vi "Przelicz ROS-a.vi"(7 "Vlin multiply":dbl, 8 "angular":dbl format="%#_13g", 9 "linear":dbl format="%#_13g", 10 "Enum":enum16{"LABVIEW", "ROS"}(ring), 11 "szablon CMD_VEL":T1) -> (3 "ROS data converted":cluster{dbl, dbl})   [LabVIEW 2015]
panel:
  in  "ROS data":T2
  out "axes":sgl[](array[numeric])
  out "buttons":i32[](array[numeric])
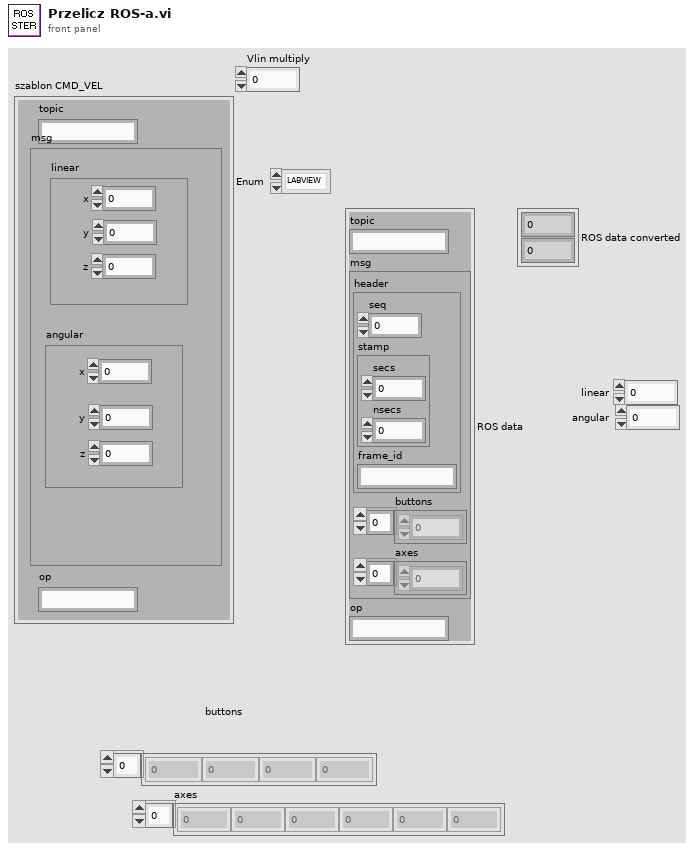
[diagram p1: front panel]
types:
  T1 = cluster{"topic":string, "msg":cluster{"linear":cluster{"x":dbl, "y":dbl, "z":dbl}, "angular":cluster{"x":dbl, "y":dbl, "z":dbl}}, "op":string}
  T2 = cluster{"topic":string, "msg":cluster{"header":cluster{"seq":u32, "stamp":cluster{"secs":u32, "nsecs":i32}, "frame_id":string}, "buttons":i32[], "axes":sgl[]}, "op":string}
  T3 = cluster{"linear":cluster{"x":dbl, "y":dbl, "z":dbl}, "angular":cluster{"x":dbl, "y":dbl, "z":dbl}}
  T4 = cluster{"header":cluster{"seq":u32, "stamp":cluster{"secs":u32, "nsecs":i32}, "frame_id":string}, "buttons":i32[], "axes":sgl[]}
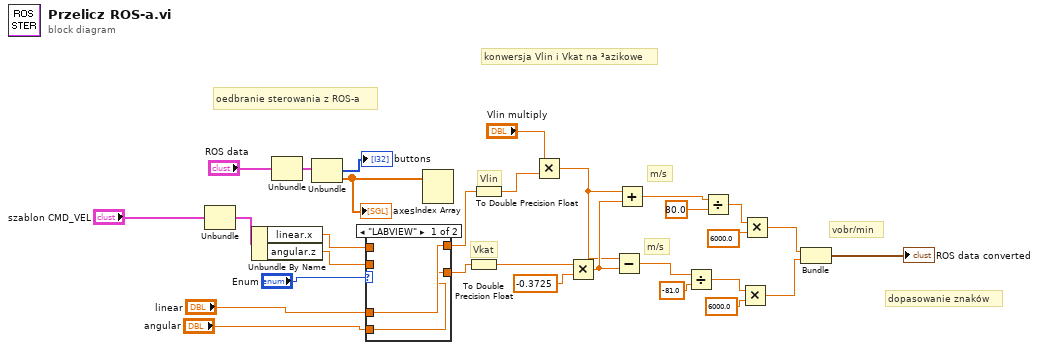
[diagram p0: block diagram]
diagram:
  # "konwersja Vlin i Vkat na ³azikowe"
  # "oedbranie sterowania z ROS-a"
  # "dopasowanie znaków"
  # "vobr/min"
  # "m/s"
  # "m/s"
  # "Vkat"
  # "Vlin"
  n1 = Unbundle("szablon CMD_VEL") -> ("msg"=w11:T3)  [unwired: 2 out]
  n2 = Unbundle By Name(w11) -> ("linear.x"=w10:dbl, "angular.z"=w9:dbl)
  n3 = Unbundle("ROS data") -> ("msg"=w28:T4)  [unwired: 2 out]
  n4 = Unbundle(w28) -> ("buttons"=→"buttons":i32[], "axes"=w25:sgl[])  [unwired: 1 out]
  "axes" <- w25
  n5 = case shown="\"LABVIEW\"" "Enum" {
    tunnel: w10 -> [_ w34]
    tunnel: w9 -> [_ w33]
    tunnel: [w32 w34] -> w8
    tunnel: [w31 w33] -> w7
    tunnel: "linear" -> [w32 _]
    tunnel: "angular" -> [w31 _]
    frame "LABVIEW" {
    }
    frame "ROS" {
    }
  }
  n6 = Index Array(array=w25) -> ()  [unwired: 2 in, 2 out]
  n7 = To Double Precision Float(number=w7) -> (double precision float=w16:dbl)
  n8 = To Double Precision Float(number=w8) -> (double precision float=w3:dbl)
  n9 = Multiply(x="Vlin multiply", y=w3) -> (x*y=w2:dbl)
  n10 = Multiply(x=w16, y=-0.3725) -> (x*y=w29:dbl)
  n11 = Subtract(x=w2, y=w29) -> (x-y=w20:dbl)
  n12 = Add(x=w2, y=w29) -> (x+y=w21:dbl)
  n13 = Divide(x=w20, y=-81.0) -> (x/y=w18:dbl)
  n14 = Divide(x=w21, y=80.0) -> (x/y=w19:dbl)
  n15 = Multiply(x=w18, y=6000.0) -> (x*y=w14:dbl)
  n16 = Multiply(x=w19, y=6000.0) -> (x*y=w15:dbl)
  n17 = Bundle(w15, w14) -> (→"ROS data converted":cluster{dbl, dbl})  [unwired: 1 in]
